vi "Build Preview.vi"(7 "Ambient":dbl, 8 "error in (no error)":errorcluster, 9 "Start Temp":dbl, 10 "Start Time":dbl, 11 "Time Step in":refnum<class "Time Step.lvclass">) -> (0 "error out":errorcluster, 1 "End Temp":dbl, 2 "End Time":dbl, 3 "Time Step out":refnum<class "Time Step.lvclass">, 4 "Step Plot Data":cluster{"Time":dbl[], "Value":dbl[]})   [LabVIEW 2018, in "Temp Recipe.lvlib" / "Time Step.lvclass"]
uses:
  Time Step.lvclass
  Time Step.lvclass/Time Step.ctl
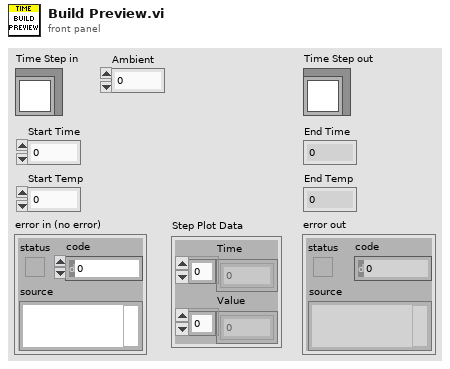
[diagram p1: front panel]
types:
  T1 = typedef "Temp Recipe.lvlib/Time Step.lvclass/Ref Data.ctl" = cluster{"Delay Time (S)":dbl}
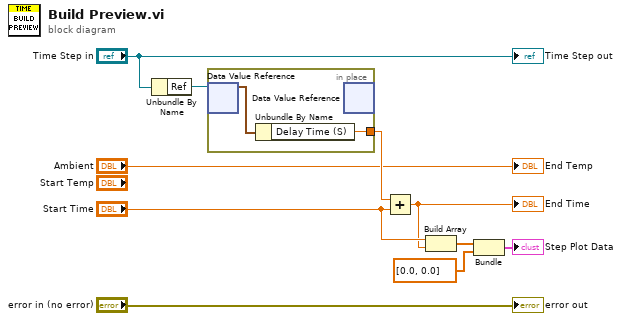
[diagram p0: block diagram]
diagram:
  n1 = Unbundle By Name("Time Step in") -> ("Ref"=w10:refnum<data-value>)
  n2 = in-place {
    in-place-border: [w11] -> w7
    n3 = in-place-dvr #1(w10) -> (w12:T1)  [unwired: 1 out]
    n4 = Unbundle By Name(w12) -> ("Delay Time (S)"=w11:dbl)
    n5 = in-place-dvr #1() -> ()  [unwired: 1 in, 2 out]
  }
  n6 = Add(x=w7, y="Start Time") -> (x+y=w6:dbl)
  "End Time" <- w6
  n7 = Build Array("Start Time", w6) -> (w5:dbl[])
  n8 = Bundle(w5, "appended array"=dbl[] [0.0, 0.0]) -> (→"Step Plot Data":cluster{dbl[], "appended array":dbl[]})  [unwired: 1 in]
  "error out" <- "error in (no error)"
  "Time Step out" <- "Time Step in"
  "End Temp" <- "Ambient"
